vi "CFTS-Is Advanced User.vi"(1 "Experimenter":string) -> (0 "Advanced user":bool)   [LabVIEW 2020]
uses:
  epl-vi-lib/Utility VIs/File IO VIs/Configuration File Wrapper VIs/Config-Read Key (string).vi
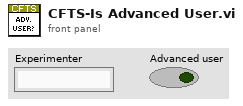
[diagram p1: front panel]
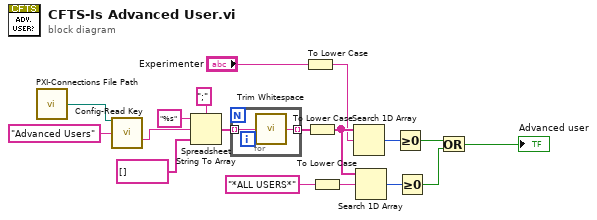
[diagram p0: block diagram]
diagram:
  n1 = call "PXI-Connections File Path.vi"() -> ("Path"=w2:path)  [unwired: 1 in]
  n2 = call-poly "Config-Read Key.vi"("configuration file path"=w2, "key"="Advanced Users") -> ("value"=w1:string)  [unwired: 10 in, 3 out]
  n3 = Spreadsheet String To Array(delimiter (Tab)=";", format string="%s", spreadsheet string=w1, array type (2D Dbl)=string[] []) -> (array=w10:string[])
  n4 = for {
    tunnel: w10 -> [w20] mode=indexing
    tunnel: [w19] -> w11 mode=indexing
    n5 = call <vilib>:"Trim Whitespace.vi"("string"=w20) -> ("trimmed string"=w19:string)  [unwired: 1 in]
  }
  n6 = To Lower Case(string="Experimenter") -> (all lower case string=w12:string)
  n7 = To Lower Case(string=w11) -> (all lower case string=w13:string[])
  n8 = To Lower Case(string="*ALL USERS*" ("element")) -> (all lower case string=w17:string)
  n9 = Search 1D Array(1D array=w13, element=w12) -> (index of element=w8:i32)  [unwired: 1 in]
  n10 = Search 1D Array(1D array=w13, element=w17) -> (index of element=w14:i32)  [unwired: 1 in]
  n11 = Greater Or Equal To 0?(x=w8) -> (x >= 0?=w9:bool)
  n12 = Greater Or Equal To 0?(x=w14) -> (x >= 0?=w15:bool)
  n13 = Or(x=w9, y=w15) -> (x .or. y?=→"Advanced user":bool)
